vi "Settings UI.vi"(11 "Settings In":T1={"Step Values"=[], "Only Execute When Test Running"=TRUE, "Reset Sequence When Test Starts"=TRUE, "Current Sequence ID"=0, "Total Iterations"=0, "Last Timestamp"=0.0, "Number of Sequence Steps"=0, "Num of Analog Channels"=0, "Num of Digital Channels"=0, "Delay Before Starting Sequence"=0.0, "Changed"=FALSE}) -> ()   [LabVIEW 2020, in "Sequencer with Output Values.lvlib" / "Sequencer with Output Values.lvclass"]
uses:
  Sequencer with Output Values.lvclass
  Params.ctl
  Step Settings.ctl
  Tree Manager/Tree Manager Mode.ctl
  Tree Manager/Control Refs.ctl
  Global Strings.vi
panel:
  out "Current Settings JSON String":string
  out "Current Settings":T1={"Step Values"=[], "Only Execute When Test Running"=TRUE, "Reset Sequence When Test Starts"=TRUE, "Current Sequence ID"=0, "Total Iterations"=0, "Last Timestamp"=0.0, "Number of Sequence Steps"=0, "Num of Analog Channels"=0, "Num of Digital Channels"=0, "Delay Before Starting Sequence"=0.0, "Changed"=FALSE}
  in  "Stop":bool
  in  "Close":bool
  in  "Apply":bool
  out "Channel Values Preview":waveform(dbl)[](graph)
  out "Setting Description":string
  in  "Tab Control":enum32{"Numeric", "String", "Bool", "Enum"}(tab)
  in  "Numeric":dbl min=1.0 max=100.0 step=1.0
  in  "String":string
  in  "Boolean":u16(ring) items=["False", "True"]
  in  "Ring":u16(ring) items=["Wait for end of step", "Repeat channel values"]
  in  "Settings Tree":string(tree) caption="Settings"
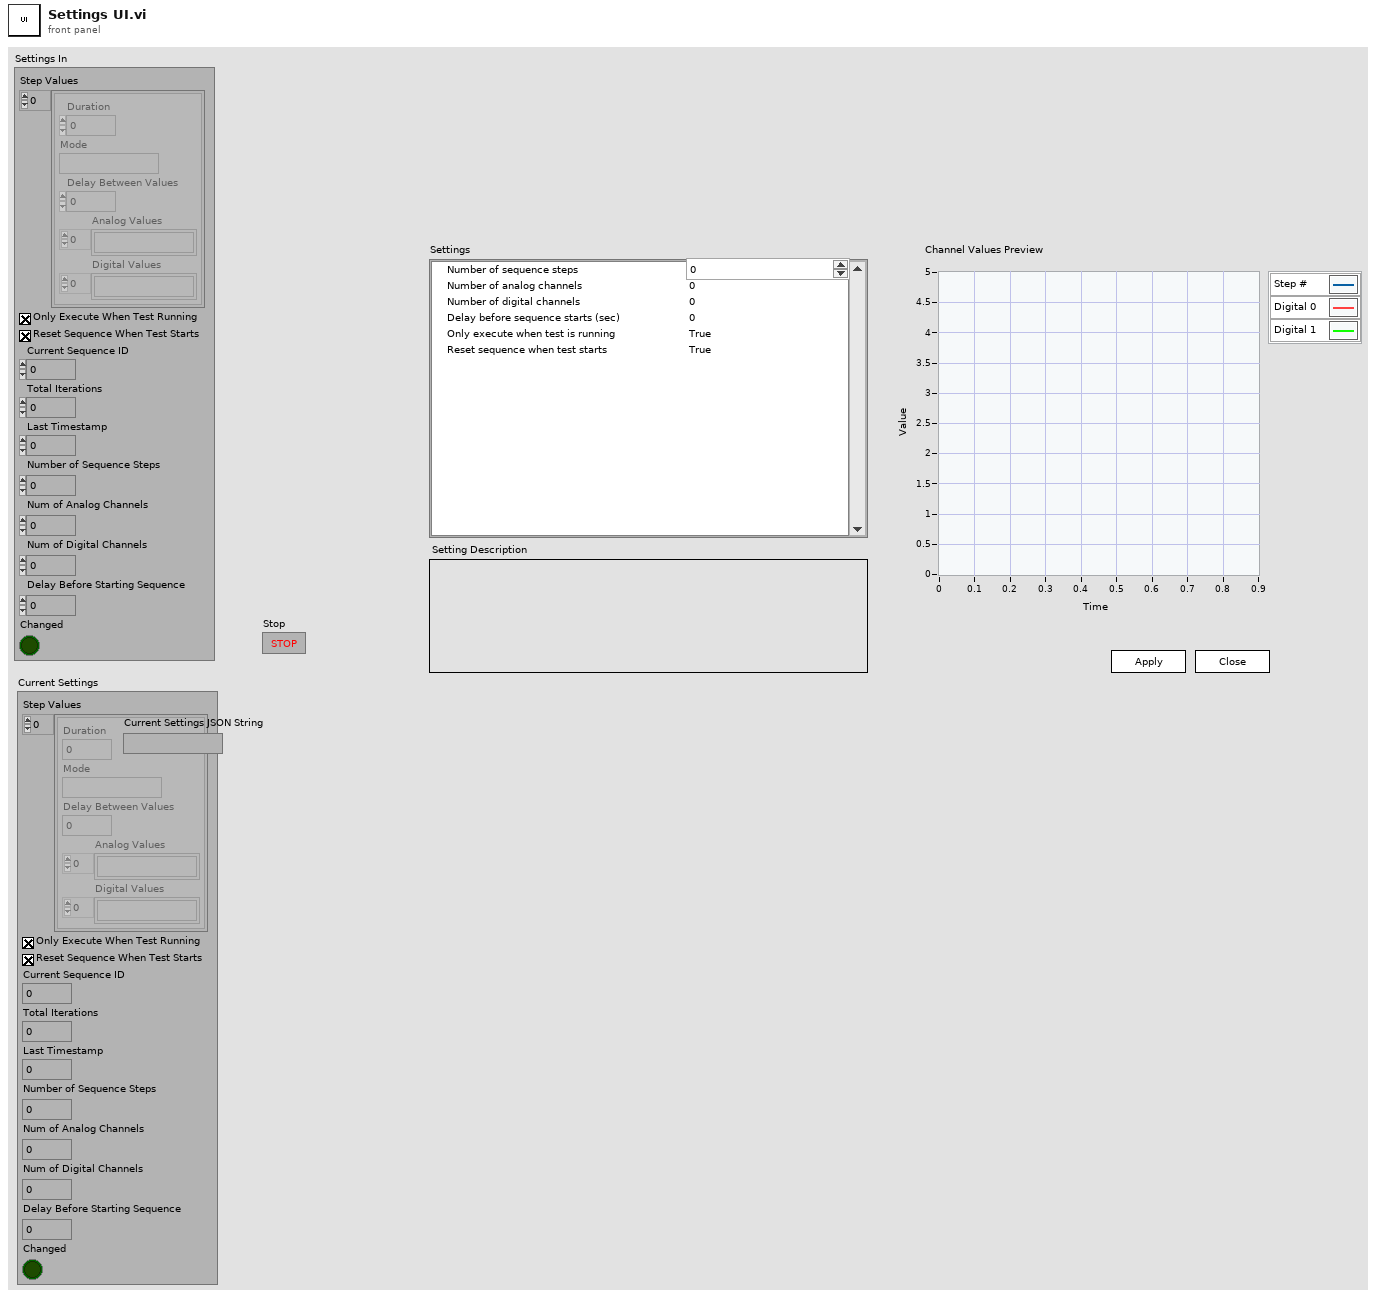
[diagram p1: front panel]
types:
  T1 = typedef "Sequencer with Output Values.lvlib/Sequencer with Output Values.lvclass/Params.ctl" = cluster{"Step Values":T2[], "Only Execute When Test Running":bool, "Reset Sequence When Test Starts":bool, "Current Sequence ID":u32, "Total Iterations":u32, "Last Timestamp":dbl, "Number of Sequence Steps":i32, "Num of Analog Channels":i32, "Num of Digital Channels":i32, "Delay Before Starting Sequence":dbl, "Changed":bool}
  T2 = typedef "Sequencer with Output Values.lvlib/Sequencer with Output Values.lvclass/Step Settings.ctl" = cluster{"Duration":dbl, "Mode":string, "Delay Between Values":dbl, "Analog Values":string[], "Digital Values":string[]}
  T3 = typedef "Sequencer with Output Values.lvlib/Sequencer with Output Values.lvclass/Tree Manager Mode.ctl" = enum16{"Init", "Tree Change", "Value Change"}
  T4 = enum32{"Invalid", "Standard", "Closed", "Hidden", "Minimized", "Maximized"}
  T5 = typedef "Sequencer with Output Values.lvlib/Sequencer with Output Values.lvclass/Control Refs.ctl" = cluster{"Tree Ref":refnum<vi>, "Tab Control":refnum<vi>, "Numeric":refnum<vi>, "String":refnum<vi>, "Boolean":refnum<vi>, "Enum":refnum<vi>, "Description":refnum<vi>}
  T6 = typedef "LVNodeAndColumnTypeDef.ctl" = cluster{"Node":string, "Column":i32}
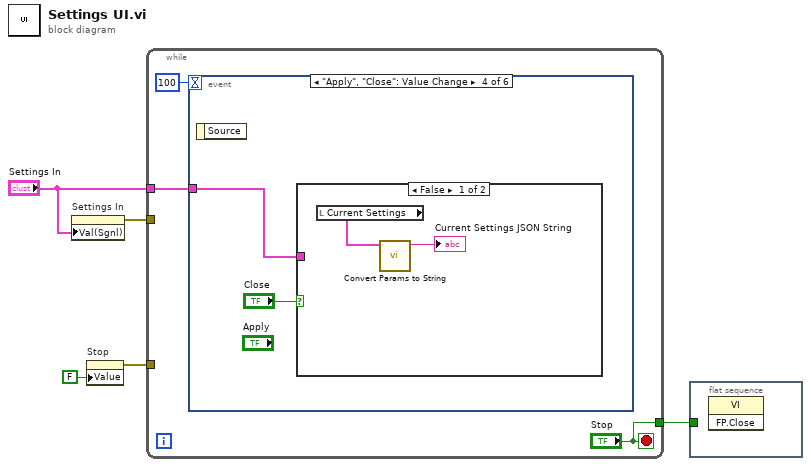
[diagram p0: block diagram]
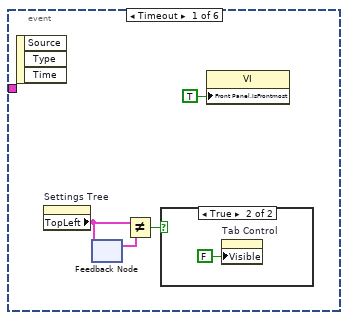
[diagram p2: hidden frame]
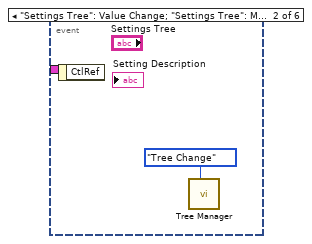
[diagram p4: hidden frame]
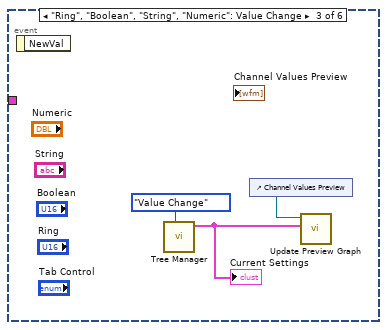
[diagram p5: hidden frame]
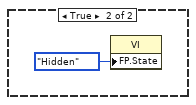
[diagram p6: hidden frame]
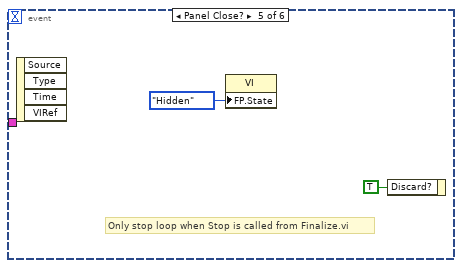
[diagram p7: hidden frame]
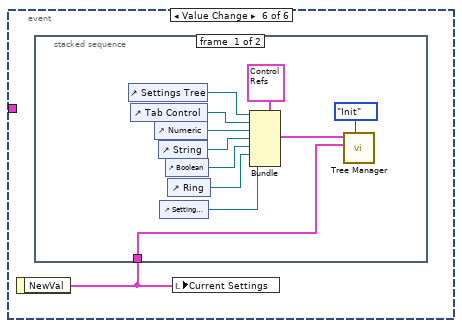
[diagram p8: hidden frame]
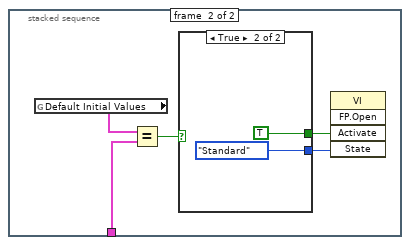
[diagram p9: hidden frame]
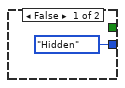
[diagram p10: hidden frame]
diagram:
  n1 = property on="Settings In" class="Clust (strict)"("Val(Sgnl)"="Settings In") -> (error out=w4:errorcluster)  [unwired: 2 in, 1 out]
  n2 = property on="Stop" class="Bool (strict)"("Value"=FALSE ("Stop")) -> (error out=w2:errorcluster)  [unwired: 2 in, 1 out]
  n3 = while {
    tunnel: "Settings In" -> [w7]
    tunnel: w4 -> [_]
    tunnel: w2 -> [_]
    tunnel: ["Stop"] -> w1
    stop <- "Stop" stop-if-true
    n4 = event shown="[3] \"Apply\", \"Close\": Value Change" {
      selector: _ -> [_ _ _ _ _ _]
      dyn-events: _ -> [_ _ _ _ _ _]
      timeout: 100 -> [_ _ _ _ _ _]
      tunnel: w7 -> [_ _ _ w18 _ _]
      event Timeout {
        n5 = event-data() -> ()  [unwired: 1 in, 3 out]
        n6 = property on="Settings Tree" class="Tree (strict)"() -> ("TopLeft"=w12:T6)  [unwired: 2 in, 2 out]
        n7 = feedback-in #1(w12) -> ()
        n8 = feedback #1() -> (w11:T6)  [unwired: 1 in]
        n9 = Not Equal?(x=w12, y=w11) -> (x != y?=w10:bool)
        n10 = case shown="True" w10 {
          frame False {
          }
          frame True {
            n11 = property on="Tab Control" class="TabCtl (strict)"("Visible"=FALSE) -> ()  [unwired: 2 in, 2 out]
          }
        }
        n12 = property class="VI"("Front Panel.IsFrontmost"=TRUE ("Front Panel Window:Is Frontmost")) -> ()  [unwired: 2 in, 2 out]
      }
      event "Settings Tree": Value Change; "Settings Tree": Mouse Down {
        n13 = event-data() -> ()  [unwired: 1 in, 1 out]
        n14 = call "Tree Manager.vi"("Mode"=Tree_Manager_Mode."Tree Change") -> ()  [unwired: 10 in, 1 out]
      }
      event "Ring", "Boolean", "String", "Numeric": Value Change {
        n15 = event-data() -> ()  [unwired: 1 in, 1 out]
        n16 = call "Tree Manager.vi"("Mode"=Tree_Manager_Mode."Value Change") -> ("Settings Out"=w16:T1)  [unwired: 10 in]
        "Current Settings" <- w16
        n17 = control-ref of="Channel Values Preview"() -> (w15:refnum<vi>)
        n18 = call "Update Preview Graph.vi"("Settings In"=w16, "Graph Preview Ref"=w15) -> ()  [unwired: 10 in]
      }
      event "Apply", "Close": Value Change {
        n19 = event-data() -> ()  [unwired: 1 in, 1 out]
        n20 = case shown="False" "Close" {
          tunnel: w18 -> [_ _]
          frame False {
            n21 = local read "Current Settings"() -> (w21:T1)
            n22 = call "Convert Params to String.vi"("Settings"=w21) -> ("String out"=→"Current Settings JSON String":string)  [unwired: 10 in]
          }
          frame True {
            n23 = property class="VI"("FP.State"=T4."Hidden" ("Front Panel Window:State")) -> ()  [unwired: 2 in, 2 out]
          }
        }
      }
      event Panel Close? {
        # "Only stop loop when Stop is called from Finalize.vi"
        n24 = event-data() -> ()  [unwired: 1 in, 4 out]
        n25 = property class="VI"("FP.State"=T4."Hidden" ("Front Panel Window:State")) -> ()  [unwired: 2 in, 2 out]
        n26 = event-data("Discard?"=TRUE) -> ()  [unwired: 1 in, 1 out]
      }
      event Value Change {
        n27 = event-data() -> ("NewVal"=w25:T1)  [unwired: 1 in]
        n28 = stacked-sequence {
          tunnel: w25 -> [w26 w38]
          frame #0 {
            n29 = control-ref of="Settings Tree"() -> (w36:refnum<vi>)
            n30 = control-ref of="Tab Control"() -> (w35:refnum<vi>)
            n31 = control-ref of="Numeric"() -> (w34:refnum<vi>)
            n32 = control-ref of="String"() -> (w33:refnum<vi>)
            n33 = control-ref of="Setting Description"() -> (w29:refnum<vi>)
            n34 = control-ref of="Boolean"() -> (w32:refnum<vi>)
            n35 = control-ref of="Ring"() -> (w31:refnum<vi>)
            n36 = Bundle(cluster=T5 {"Tree Ref"=refnum, "Tab Control"=refnum, "Numeric"=refnum, "String"=refnum, "Boolean"=refnum, "Enum"=refnum, "Description"=refnum} ("Init Refs"), "Tree Ref"=w36, "Tab Control"=w35, "Numeric"=w34, "String"=w33, "Boolean"=w32, "Enum"=w31, "Description"=w29) -> (w30:T5)
            n37 = call "Tree Manager.vi"("Mode"=Tree_Manager_Mode."Init", "Settings In"=w26, "Init Refs"=w30) -> ()  [unwired: 8 in, 1 out]
          }
          frame #1 {
            n38 = global read "Global Strings.vi" "Default Initial Values"() -> (w37:T1)
            n39 = Equal?(x=w37, y=w38) -> (x = y?=w41:bool)
            n40 = case shown="True" w41 {
              tunnel: [_ TRUE ("Activate?")] -> w40
              tunnel: [T4."Hidden" ("State") T4."Standard" ("State")] -> w39
              frame False {
              }
              frame True {
              }
            }
            n41 = invoke class="VI" method="FP.Open"("Activate"=w40, "State"=w39) -> ()  [unwired: 3 in, 5 out]
          }
        }
        n42 = local write "Current Settings"(w25) -> ()
      }
    }
  }
  n43 = flat-sequence {
    tunnel: w1 -> [_]
    frame #0 {
      n44 = invoke class="VI" method="FP.Close"() -> ()  [unwired: 3 in, 3 out]
    }
  }
